vi "GEA2 Script_Parse ERD Write.vi"(0 "Data":string, 11 "Error In":errorcluster) -> (6 "GEA Inputs":T1 {"Destination" format="%.0x"; "Source" format="%.0x"}, 8 "Write ERD List":T2[](array[typedef]) {"ERD Number" format="%.0x"}, 15 "Error Out":errorcluster)   [LabVIEW 2023]
uses:
  LabVIEW GEA2 Toolkit/GEA3/type defs/ERD Write Data In.ctl
  LabVIEW GEA2 Toolkit/GEA3/type defs/Data Type.ctl
  LabVIEW GEA2 Toolkit/GEA3/type defs/Source_Destination.ctl
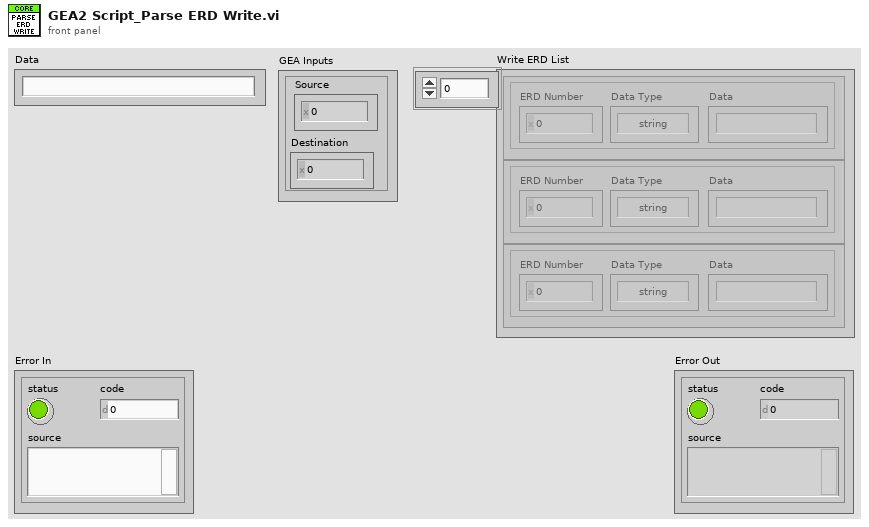
[diagram p1: front panel]
types:
  T1 = typedef "Source_Destination.ctl" = cluster{"Source":u8, "Destination":u8}
  T2 = typedef "ERD Write Data In.ctl" = cluster{"ERD Number":u16, "Data Type":T3, "Data":string}
  T3 = typedef "Data Type.ctl" = enum16{"string", "boolean", "uint8_t", "uint16_t", "uint32_t", "uint64_t", "int8_t", "int16_t", "int32_t", "int64_t"}
  T4 = enum16{"string", "boolean", "uint8_t", "uint16_t", "uint32_t"}
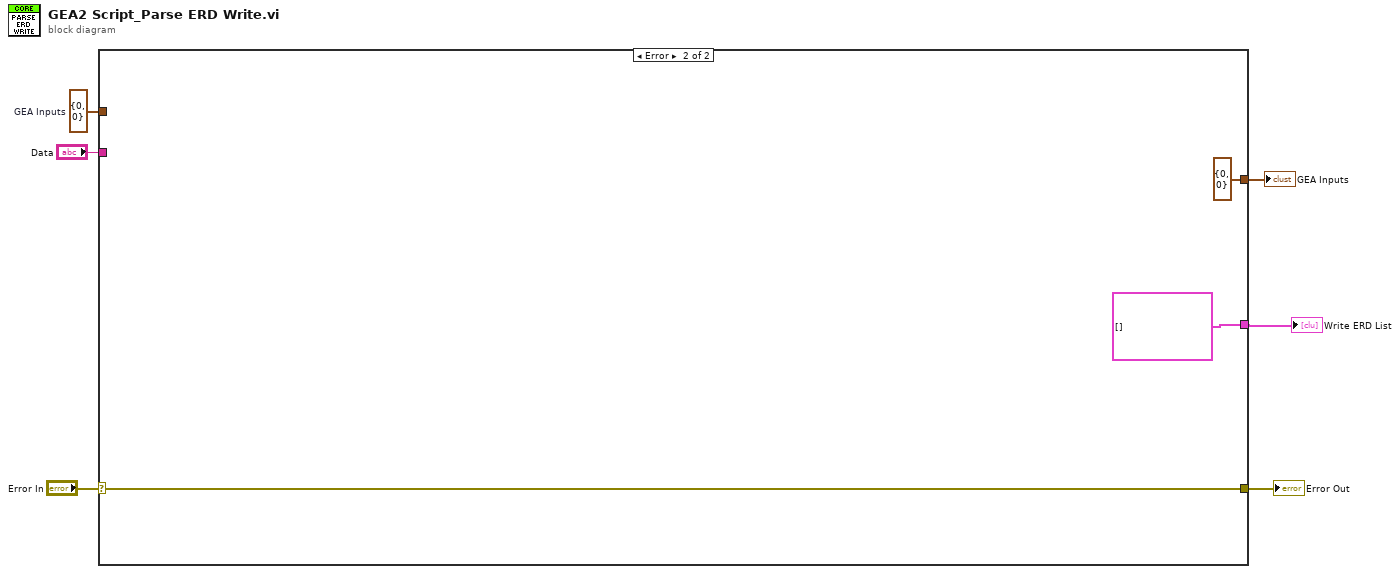
[diagram p0: block diagram]
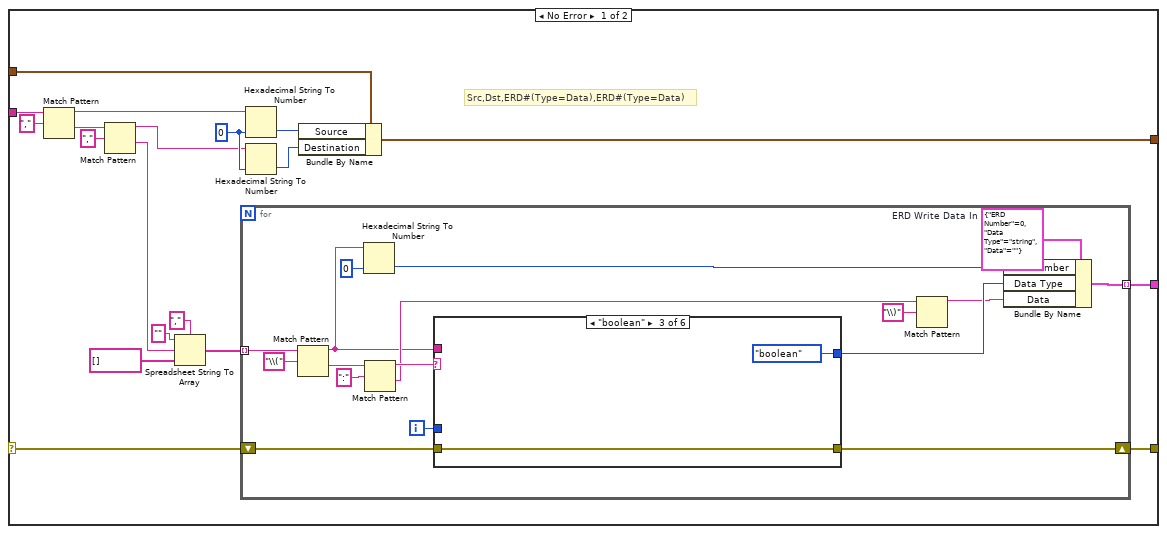
[diagram p2: hidden frame]
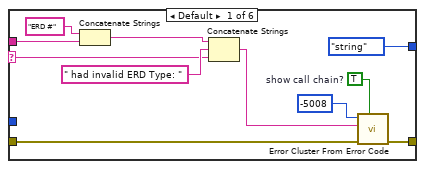
[diagram p3: hidden frame]
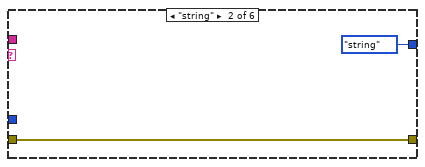
[diagram p4: hidden frame]
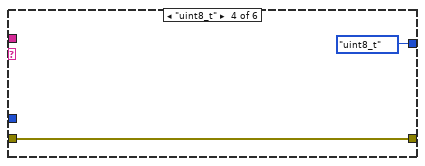
[diagram p5: hidden frame]
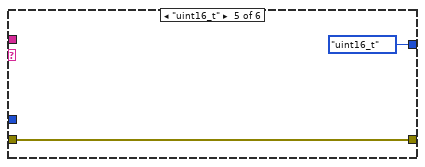
[diagram p6: hidden frame]
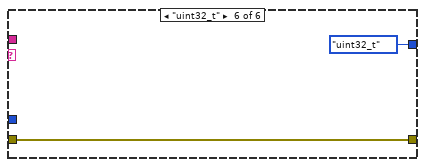
[diagram p7: hidden frame]
diagram:
  w5 = T1 {"Source"=0, "Destination"=0}  # GEA Inputs
  n1 = case shown="Error" "Error In" {
    selector: "Error In" -> [w13 w66]
    tunnel: "Data" -> [w25 _]
    tunnel: w5 -> [w16 _]
    tunnel: [w15 T1 {"Source"=0, "Destination"=0} ("GEA Inputs")] -> w4
    tunnel: [w14 T2[] []] -> w1
    tunnel: [w12 w66] -> w2
    frame No Error {
      w19 = u8 0
      # "Src,Dst,ERD#(Type=Data),ERD#(Type=Data)"
      n2 = Match Pattern(string=w25, regular expression=",") -> (before substring=w22:string, after substring=w21:string)  [unwired: 1 in, 2 out]
      n3 = Match Pattern(string=w21, regular expression=",") -> (before substring=w18:string, after substring=w10:string)  [unwired: 1 in, 2 out]
      n4 = Spreadsheet String To Array(delimiter (Tab)=",", format string="", spreadsheet string=w10, array type (2D Dbl)=string[] []) -> (array=w8:string[])
      n5 = for {
        tunnel: [w39] -> w14 mode=indexing
        shift-right: [w32] -> w12
        shift-left: w13 -> [w33]
        tunnel: w8 -> [w29] mode=indexing
        i -> [w28]
        w26 = T2 {"ERD Number"=0, "Data Type"=enum."string", "Data"=""}  # ERD Write Data In
        n6 = Match Pattern(string=w29, regular expression="\\(") -> (before substring=w27:string, after substring=w34:string)  [unwired: 1 in, 2 out]
        n7 = Hexadecimal String To Number(string=w27, default (0uL)=u16 0 ("ERD Number")) -> (number=w41:u16)  [unwired: 1 in, 1 out]
        n8 = Match Pattern(string=w34, regular expression=":") -> (before substring=w31:string, after substring=w30:string)  [unwired: 1 in, 2 out]
        n9 = case shown="\"boolean\"" w31 {
          selector: w31 -> [w47 _ _ _ _ _]
          tunnel: [T4."string" ("Data Type") T4."string" ("Data Type") T4."boolean" ("Data Type") T4."uint8_t" ("Data Type") T4."uint16_t" ("Data Type") T4."uint32_t" ("Data Type")] -> w37
          tunnel: w33 -> [w52 w54 w56 w58 w60 w62]
          tunnel: [w51 w54 w56 w58 w60 w62] -> w32
          tunnel: w28 -> [_ _ _ _ _ _]
          tunnel: w27 -> [w44 _ _ _ _ _]
          frame Default {
            w49 = TRUE  # show call chain?
            n10 = Concatenate Strings("ERD #", w44) -> (w43:string)
            n11 = Concatenate Strings(w43, " had invalid ERD Type: " ("error message (\"\")"), w47) -> (w46:string)
            n12 = call <vilib>:"Error Cluster From Error Code.vi"("show call chain? (False)"=w49, "error in (no error)"=w52, "error message (\"\")"=w46, "error code (0)"=-5008) -> ("error out"=w51:errorcluster)  [unwired: 5 in]
          }
          frame "string" {
          }
          frame "boolean" {
          }
          frame "uint8_t" {
          }
          frame "uint16_t" {
          }
          frame "uint32_t" {
          }
        }
        n13 = Match Pattern(string=w30, regular expression="\\)") -> (before substring=w35:string)  [unwired: 1 in, 3 out]
        n14 = Bundle By Name(cluster=w26, "ERD Number"=w41, "Data Type"=w37, "Data"=w35) -> (w39:T2)
      }
      n15 = Hexadecimal String To Number(string=w22, default (0uL)=w19) -> (number=w20:u8)  [unwired: 1 in, 1 out]
      n16 = Hexadecimal String To Number(string=w18, default (0uL)=w19) -> (number=w17:u8)  [unwired: 1 in, 1 out]
      n17 = Bundle By Name(cluster=w16, "Source"=w20, "Destination"=w17) -> (w15:T1)
    }
    frame Error {
    }
  }
  "Write ERD List" <- w1
  "GEA Inputs" <- w4
  "Error Out" <- w2
